vi "Wrapper for JKI Parse State Queue.vi"(4 "pause execution":bool, 6 "cancel execution":bool, 8 "error in (no error)":errorcluster, 11 "State Queue":string) -> (1 "Arguments":string, 2 "Current State":string, 3 "Remaining States":string)   [LabVIEW 2017]
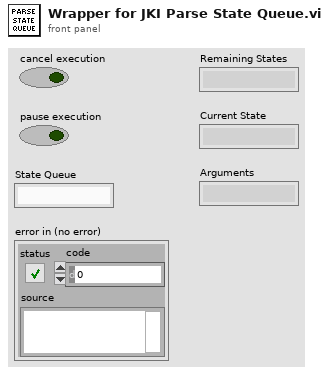
[diagram p1: front panel]
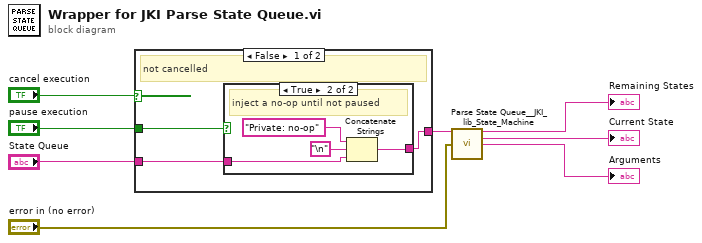
[diagram p0: block diagram]
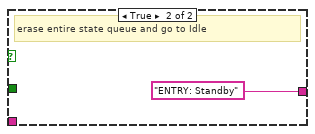
[diagram p3: hidden frame]
diagram:
  n1 = case shown="False" "cancel execution" {
    tunnel: "State Queue" -> [w11 _]
    tunnel: [w10 "ENTRY: Standby"] -> w7
    tunnel: "pause execution" -> [w9 _]
    frame False {
      # "not cancelled"
      n2 = case shown="True" w9 {
        tunnel: w11 -> [w12 w14]
        tunnel: [w12 w13] -> w10
        frame False {
          # "not paused"
        }
        frame True {
          # "inject a no-op until not paused"
          n3 = Concatenate Strings("Private: no-op", "\n", w14) -> (w13:string)
        }
      }
    }
    frame True {
      # "erase entire state queue and go to Idle"
    }
  }
  n4 = call <vilib>:"Parse State Queue__JKI_lib_State_Machine.vi"("State Queue"=w7, "Error In (no error)"="error in (no error)") -> ("Remaining States"=→"Remaining States":string, "Current State"=→"Current State":string, "Arguments"=→"Arguments":string)  [unwired: 11 in]
